vi "Channel_Name_Options.vi"(0 "All Channel Names":string[](array[string]), 1 "Data string":string, 2 "Ignore When":string[][](array[string]), 3 "Reading Filename":path, 5 "Template Names":string[](array[string]), 7 "Channels OK":bool[](array[boolean]), 9 "Start of data (bytes)":i32, 11 "Maths In":string[](array[string]), 12 "Name Options In":string[][](array[string]), 13 "Filetype":string) -> (4 "Channels to find":string[](array[string]), 6 "Valid Channel Options":string[][](array[string]), 15 "Name Options Out":string[][](array[string]))   [LabVIEW 2010]
uses:
  Results_plotter_Global.vi
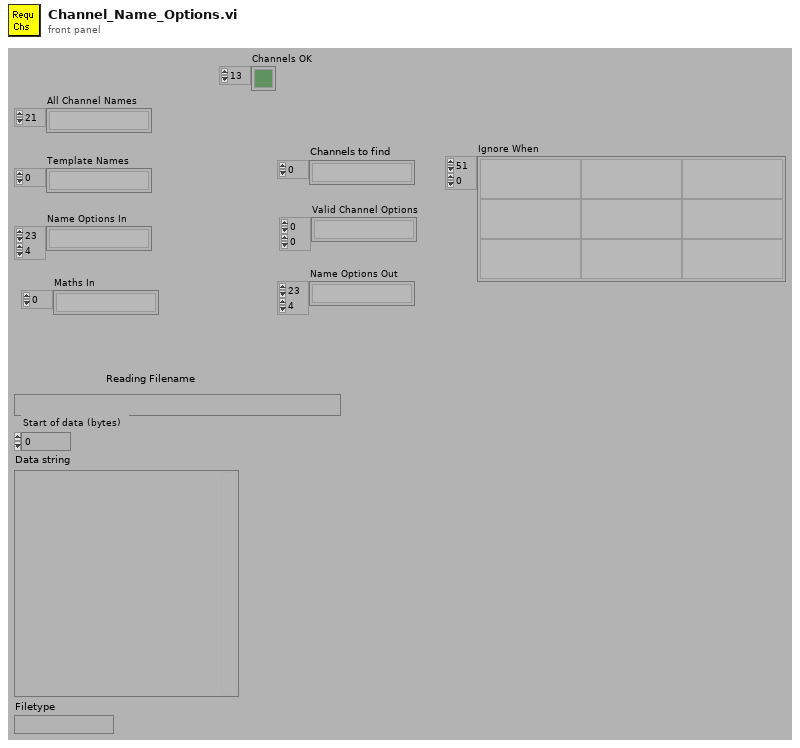
[diagram p1: front panel]
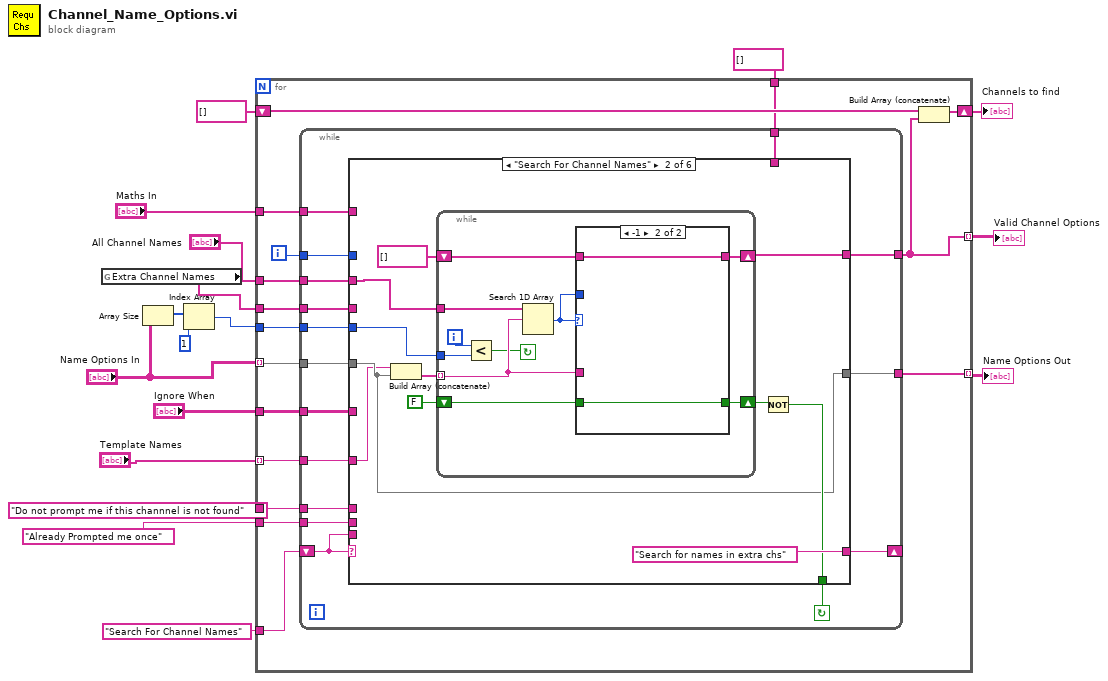
[diagram p0: block diagram]
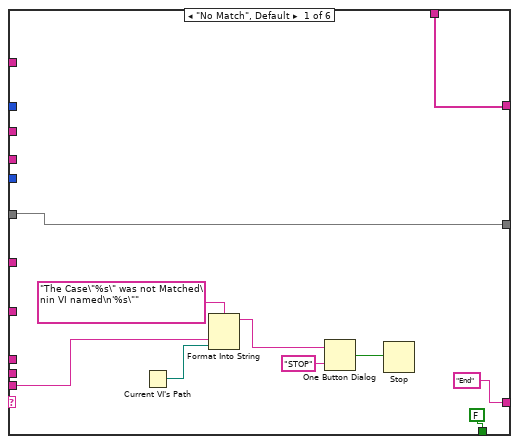
[diagram p2: hidden frame]
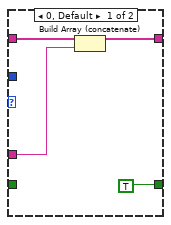
[diagram p3: hidden frame]
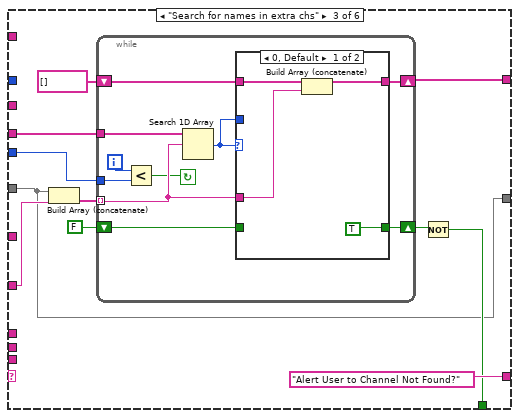
[diagram p4: hidden frame]
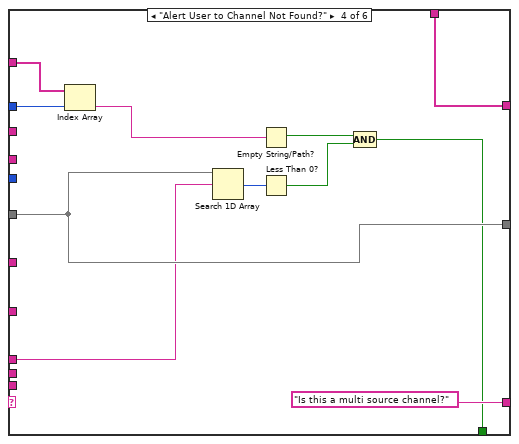
[diagram p6: hidden frame]
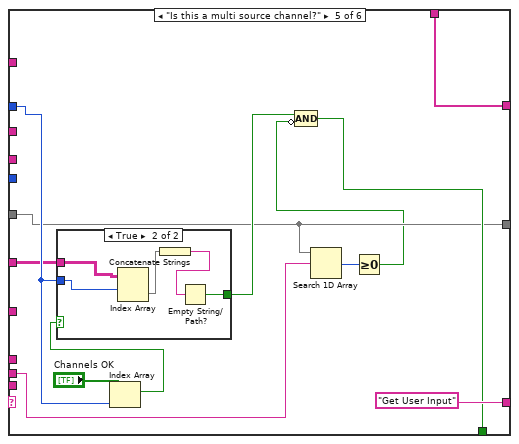
[diagram p7: hidden frame]
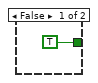
[diagram p8: hidden frame]
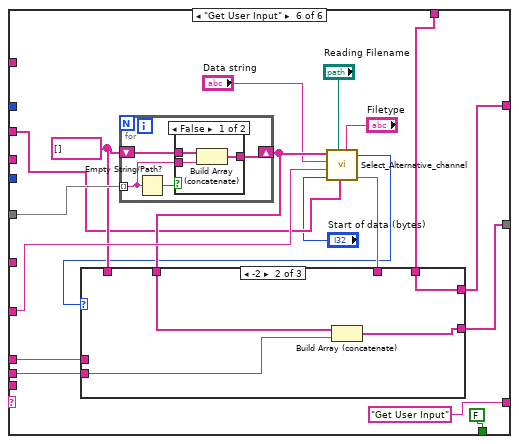
[diagram p9: hidden frame]
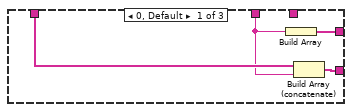
[diagram p10: hidden frame]
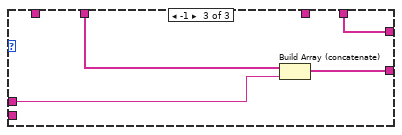
[diagram p11: hidden frame]
diagram:
  n1 = global read "Results_plotter_Global.vi" "Extra Channel Names"() -> (w4:string[])
  n2 = Array Size(array="Name Options In") -> (size(s)=w15:i32[])
  n3 = Index Array(array=w15, index=1 ("Index")) -> (element=w12:i32)
  n4 = for {
    tunnel: "All Channel Names" -> [w33]
    tunnel: "Name Options In" -> [w31] mode=indexing
    tunnel: w12 -> [w32]
    tunnel: [w22] -> w9 mode=indexing
    tunnel: "Template Names" -> [w30] mode=indexing
    tunnel: [w29] -> w17 mode=indexing
    tunnel: "Do not prompt me if this channnel is not found" -> [w28]
    tunnel: "Maths In" -> [w27]
    tunnel: "Search For Channel Names" -> [w25]
    shift-right: [w23] -> w7
    shift-left: string[] [] -> [w24]
    tunnel: string[] [] -> [w21]
    tunnel: w4 -> [w20]
    tunnel: "Already Prompted me once" -> [w19]
    tunnel: "Ignore When" -> [w18]
    i -> [w26]
    n5 = while {
      tunnel: w20 -> [w36]
      tunnel: w21 -> [w37]
      tunnel: [w38] -> w22
      tunnel: w26 -> [w39]
      tunnel: w27 -> [w41]
      tunnel: w28 -> [w42]
      tunnel: [w43] -> w29
      tunnel: w30 -> [w44]
      tunnel: w31 -> [w47]
      tunnel: w32 -> [w48]
      tunnel: w33 -> [w49]
      shift-left: w25 -> [w40]
      shift-right: [w45] -> _
      tunnel: w19 -> [w35]
      tunnel: w18 -> [w34]
      stop <- w46 continue-if-true
      n6 = case shown="\"Search For Channel Names\"" w40 {
        tunnel: w49 -> [_ w61 _ _ _ w148]
        tunnel: w48 -> [_ w70 w97 _ _ _]
        tunnel: w47 -> [w51 w62 w88 w123 w128 w160]
        tunnel: [w50 w66 w93 w114 w135 w157] -> w38
        tunnel: [FALSE w64 w91 w118 w134 FALSE] -> w46
        tunnel: ["End" "Search for names in extra chs" "Alert User to Channel Not Found?" "Is this a multi source channel?" "Get User Input" "Get User Input"] -> w45
        tunnel: w44 -> [_ w60 w90 _ _ w156]
        tunnel: [w51 w62 w88 w123 w128 w158] -> w43
        tunnel: w42 -> [_ _ _ w122 _ w144]
        tunnel: w41 -> [_ _ _ w117 _ _]
        tunnel: w40 -> [w54 _ _ _ _ _]
        tunnel: w39 -> [_ _ _ w116 w131 _]
        tunnel: w37 -> [w50 _ _ w114 w135 w151]
        tunnel: w36 -> [_ _ w87 _ _ _]
        tunnel: w35 -> [_ _ _ _ w127 w143]
        tunnel: w34 -> [_ _ _ _ w126 _]
        frame "No Match", Default {
          n7 = Current VI's Path() -> (path=w55:path)
          n8 = Format Into String(format string="The Case\"%s\" was not Matched\nin VI named\n'%s\"" ("Format String"), w54, w55) -> (resulting string=w58:string)  [unwired: 2 in, 1 out]
          n9 = One Button Dialog(message=w58, button name ("OK")="STOP") -> (true=w56:bool)
          n10 = Stop(stop? (T)=w56) -> ()
        }
        frame "Search For Channel Names" {
          n11 = Build Array (concatenate)(w60, w62) -> (w63:string[])
          n12 = while {
            shift-left: string[] [] -> [w72]
            shift-right: [w75] -> w66
            shift-left: FALSE ("index of element") -> [w73]
            shift-right: [w74] -> w65
            tunnel: w63 -> [w77] mode=indexing
            tunnel: w70 -> [w78]
            tunnel: w61 -> [w80]
            i -> [w79]
            stop <- w71 continue-if-true
            n13 = Less?(x=w79, y=w78) -> (x < y?=w71:bool)
            n14 = Search 1D Array(1D array=w80, element=w77) -> (index of element=w76:i32)  [unwired: 1 out]
            n15 = case shown="-1" w76 {
              tunnel: w77 -> [w82 _]
              tunnel: w76 -> [_ _]
              tunnel: [w83 w85] -> w75
              tunnel: [TRUE w86] -> w74
              tunnel: w73 -> [_ w86]
              tunnel: w72 -> [w84 w85]
              frame 0, Default {
                n16 = Build Array (concatenate)(w84, w82) -> (w83:string[])
              }
              frame -1 {
              }
            }
          }
          n17 = Not(x=w65) -> (.not. x?=w64:bool)
        }
        frame "Search for names in extra chs" {
          n18 = Build Array (concatenate)(w88, w90) -> (w89:string[])
          n19 = while {
            shift-left: string[] [] -> [w99]
            shift-right: [w102] -> w93
            shift-left: FALSE ("index of element") -> [w100]
            shift-right: [w101] -> w92
            tunnel: w89 -> [w104] mode=indexing
            tunnel: w97 -> [w105]
            tunnel: w87 -> [w107]
            i -> [w106]
            stop <- w98 continue-if-true
            n20 = Less?(x=w106, y=w105) -> (x < y?=w98:bool)
            n21 = Search 1D Array(1D array=w107, element=w104) -> (index of element=w103:i32)  [unwired: 1 out]
            n22 = case shown="0, Default" w103 {
              tunnel: w104 -> [w109 _]
              tunnel: w103 -> [_ _]
              tunnel: [w110 w112] -> w102
              tunnel: [TRUE w113] -> w101
              tunnel: w100 -> [_ w113]
              tunnel: w99 -> [w111 w112]
              frame 0, Default {
                n23 = Build Array (concatenate)(w111, w109) -> (w110:string[])
              }
              frame -1 {
              }
            }
          }
          n24 = Not(x=w92) -> (.not. x?=w91:bool)
        }
        frame "Alert User to Channel Not Found?" {
          n25 = Index Array(array=w117, index=w116) -> (element=w115:string)
          n26 = Search 1D Array(1D array=w123, element=w122) -> (index of element=w124:i32)  [unwired: 1 out]
          n27 = Empty String/Path?(string/path=w115) -> (empty?=w120:bool)
          n28 = Less Than 0?(x=w124) -> (x < 0?=w119:bool)
          n29 = Compound Arithmetic op=AND(w120, w119) -> (w118:bool)
        }
        frame "Is this a multi source channel?" {
          n30 = Index Array(array="Channels OK", index=w131) -> (element=w132:bool)
          n31 = case shown="True" w132 {
            tunnel: [TRUE w142] -> w133
            tunnel: w131 -> [_ w141]
            tunnel: w126 -> [_ w138]
            frame False {
            }
            frame True {
              n32 = Index Array(array=w138, index (row)=w141) -> (element=w140:string[])  [unwired: 1 in]
              n33 = Concatenate Strings(w140) -> (w139:string)
              n34 = Empty String/Path?(string/path=w139) -> (empty?=w142:bool)
            }
          }
          n35 = Search 1D Array(1D array=w128, element=w127) -> (index of element=w129:i32)  [unwired: 1 out]
          n36 = Greater Or Equal To 0?(x=w129) -> (x >= 0?=w125:bool)
          n37 = Compound Arithmetic op=AND(w133, invert w125) -> (w134:bool)
        }
        frame "Get User Input" {
          w153 = string[] []
          n38 = for {
            shift-right: [w173] -> w155
            shift-left: w153 -> [w175]
            tunnel: w160 -> [w174] mode=indexing
            n39 = Empty String/Path?(string/path=w174) -> (empty?=w176:bool)
            n40 = case shown="False" w176 {
              tunnel: w175 -> [w179 w180]
              tunnel: [w178 w180] -> w173
              tunnel: w174 -> [w177 _]
              frame False {
                n41 = Build Array (concatenate)(w179, w177) -> (w178:string[])
              }
              frame True {
              }
            }
          }
          n42 = call "Select_Alternative_channel.vi"("Filetype"="Filetype", "All Tabulated Channels"=w148, "Reading Filename"="Reading Filename", "Start of data (bytes)"="Start of data (bytes)", "Template Channel Name"=w156, "Data string"="Data string", "Previous Channels used"=w155) -> ("Choosen Channel"=w154:string, "Selected Index"=w150:i32)  [unwired: 2 out]
          n43 = case shown="-2" w150 {
            tunnel: [w164 w166 w172] -> w158
            tunnel: [w161 w168 w171] -> w157
            tunnel: w155 -> [w163 w167 w170]
            tunnel: w154 -> [w162 _ _]
            tunnel: w153 -> [_ _ _]
            tunnel: w151 -> [_ w168 w171]
            tunnel: w144 -> [_ _ w169]
            tunnel: w143 -> [_ w165 _]
            frame 0, Default {
              n44 = Build Array(w162) -> (w161:string[])
              n45 = Build Array (concatenate)(w163, w162) -> (w164:string[])
            }
            frame -2 {
              n46 = Build Array (concatenate)(w167, w165) -> (w166:string[])
            }
            frame -1 {
              n47 = Build Array (concatenate)(w170, w169) -> (w172:string[])
            }
          }
        }
      }
    }
    n48 = Build Array (concatenate)(w24, w22) -> (w23:string[])
  }
  "Name Options Out" <- w17
  "Valid Channel Options" <- w9
  "Channels to find" <- w7
